vi "Write Default Channels to File.vi"(8 "error in (no error)":errorcluster, 10 "Channels":string[](array[string]), 11 "SysDef File Path":path) -> (0 "error out":errorcluster)   [LabVIEW 2015]
uses:
  <vilib>/Utility/config.llb/Write Key (Boolean).vi
  <vilib>/Utility/config.llb/NI_LVConfig.lvlib
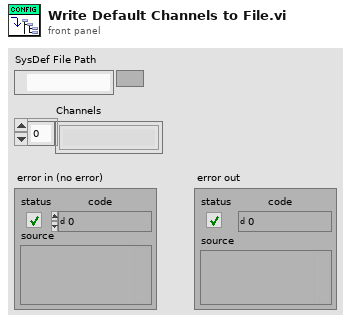
[diagram p1: front panel]
types:
  T1 = typedef "NI_LVConfig.lvlib/Config Data RefNum.ctl" = refnum<k1>
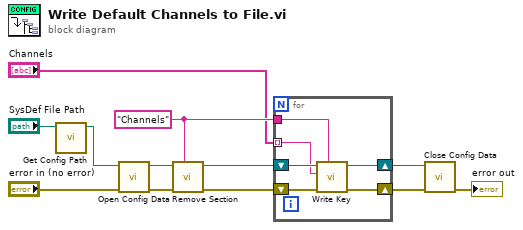
[diagram p0: block diagram]
diagram:
  w7 = "Channels" ("section")
  n1 = call "Get Config Path.vi"("Sys Def Path"="SysDef File Path") -> ("Config Path"=w3:path)  [unwired: 9 in, 1 out]
  n2 = call <vilib>:"Open Config Data.vi"("error in (no error)"="error in (no error)", "configuration file path"=w3) -> ("error out"=w2:errorcluster, "refnum"=w9:T1)  [unwired: 7 in, 1 out]
  n3 = call <vilib>:"Remove Section.vi"("section"=w7, "error in (no error)"=w2, "refnum"=w9) -> ("error out"=w5:errorcluster, "refnum out"=w10:T1)  [unwired: 6 in, 1 out]
  n4 = for {
    shift-right: [w17] -> w4
    shift-left: w5 -> [w18]
    shift-right: [w16] -> w11
    shift-left: w10 -> [w15]
    tunnel: w7 -> [w14]
    tunnel: "Channels" -> [w13] mode=indexing
    n5 = call-poly <vilib>:"Write Key.vi"("section"=w14, "error in (no error)"=w18, "key"=w13, "refnum"=w15) -> ("error out"=w17:errorcluster, "refnum out"=w16:T1)  [unwired: 5 in, 1 out]
  }
  n6 = call <vilib>:"Close Config Data.vi"("error in (no error)"=w4, "refnum"=w11) -> ("error out"=→"error out":errorcluster)  [unwired: 8 in, 1 out]
